vi "FMA1600A Initialize.vi"(7 "baud rate (9600)":u32=19200, 8 "error in (no error)":errorcluster, 11 "VISA Refnum in":refnum<visa-resource-name>) -> (0 "error out":errorcluster, 3 "VISA Refnum out":refnum<visa-resource-name>)   [LabVIEW 2016]
uses:
  <vilib>/Instr/_visa.llb/VISA Open Access Mode.ctl
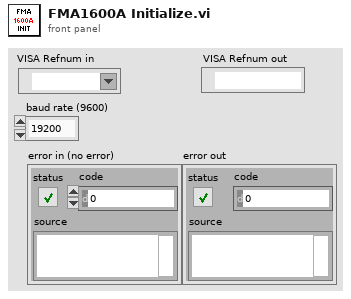
[diagram p1: front panel]
types:
  T1 = typedef "VISA Open Access Mode.ctl" = u32
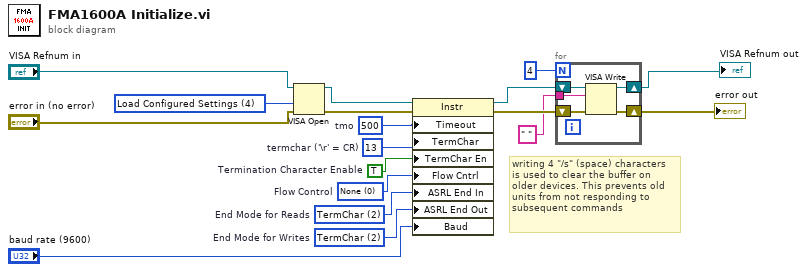
[diagram p0: block diagram]
diagram:
  w8 = T1 4 items=["VISA Defaults"=0, "Exclusive Lock"=1, "Load Configured Settings"=4] ("Access Mode")
  w9 = u32 500  # tmo
  w10 = u16 2 items=["None", "Last Bit", "TermChar", "Break"]  # End Mode for Writes
  w11 = u16 2 items=["None", "Last Bit", "TermChar"]  # End Mode for Reads
  w12 = u16 0 items=["None", "XON/XOFF", "RTS/CTS", "XON/XOFF & RTS/CTS", "DTR/DSR", "XON/XOFF & DTR/DSR"]  # Flow Control
  w13 = TRUE  # Termination Character Enable
  w14 = u8 13  # termchar ('\r' = CR)
  # "writing 4 \"/s\" (space) characters\nis used to clear the buffer on \nolder devices. This prevents old\nunits from not responding to \nsubsequent commands"
  n1 = VISA Open(access mode=w8, error in (no error)="error in (no error)", VISA resource name="VISA Refnum in") -> (VISA resource name=w7:refnum<visa-resource-name>, error out=w6:errorcluster)  [unwired: 2 in]
  n2 = property class="Instr"(reference=w7, error in=w6, "Timeout"=w9, "TermChar"=w14, "TermChar En"=w13, "Flow Cntrl"=w12, "ASRL End In"=w11, "ASRL End Out"=w10, "Baud"="baud rate (9600)") -> (reference out=w18:refnum<visa-resource-name>, error out=w17:errorcluster)
  n3 = for {
    N: 4 -> [_]
    tunnel: " " -> [w19]
    shift-right: [w20] -> w4
    shift-left: w18 -> [w21]
    shift-right: [w22] -> w3
    shift-left: w17 -> [w23]
    n4 = VISA Write(VISA resource name=w21, write buffer=w19, error in (no error)=w23) -> (VISA resource name out=w20:refnum<visa-resource-name>, error out=w22:errorcluster)  [unwired: 1 out]
  }
  "VISA Refnum out" <- w4
  "error out" <- w3
